vi "GUI - Copy.vi"() -> ()   [LabVIEW 2020]
uses:
  <vilib>/DAQmx/read.llb/DAQmx Read (Analog DBL 1Chan 1Samp).vi
  <vilib>/DAQmx/miscellaneous.llb/DAQmx Fill In Error Info.vi
  <vilib>/Utility/file.llb/Write Delimited Spreadsheet (string).vi
  <vilib>/Utility/file.llb/Write Delimited Spreadsheet (DBL).vi
  <vilib>/express/express arith-compare/Formula/XNode/ExpressFormulaBlockNode.xnode
panel:
  in  "stop":bool
  in  "Tab Control":enum32{"Overview", "Graphs"}(tab)
  out "NTU":dbl
  out "NTU":dbl
  out "NTU":dbl
  out "%":dbl
  out "L/s":dbl
  out "L/s":dbl
  in  "Gauge":bool
  in  "Coagulant Dose":bool
  in  "Switch":bool
  in  "Pump 2":bool
  in  "Pump 1":bool
  in  "UV254":bool
  in  "PID 3":bool
  in  "PID 2":bool
  in  "Valve 2":bool
  in  "Flow 2":bool
  in  "NTU 2":bool
  in  "NTU 3":bool
  in  "Flow 1":bool
  in  "Valve 1":bool
  in  "PID 1":bool
  in  "NTU 1":bool
  out "L/s":cluster{dbl[], dbl[]}[](graph)
  out "NTU":cluster{dbl[], dbl[]}[](graph)
  in  "Seconds per data point (sec)":dbl
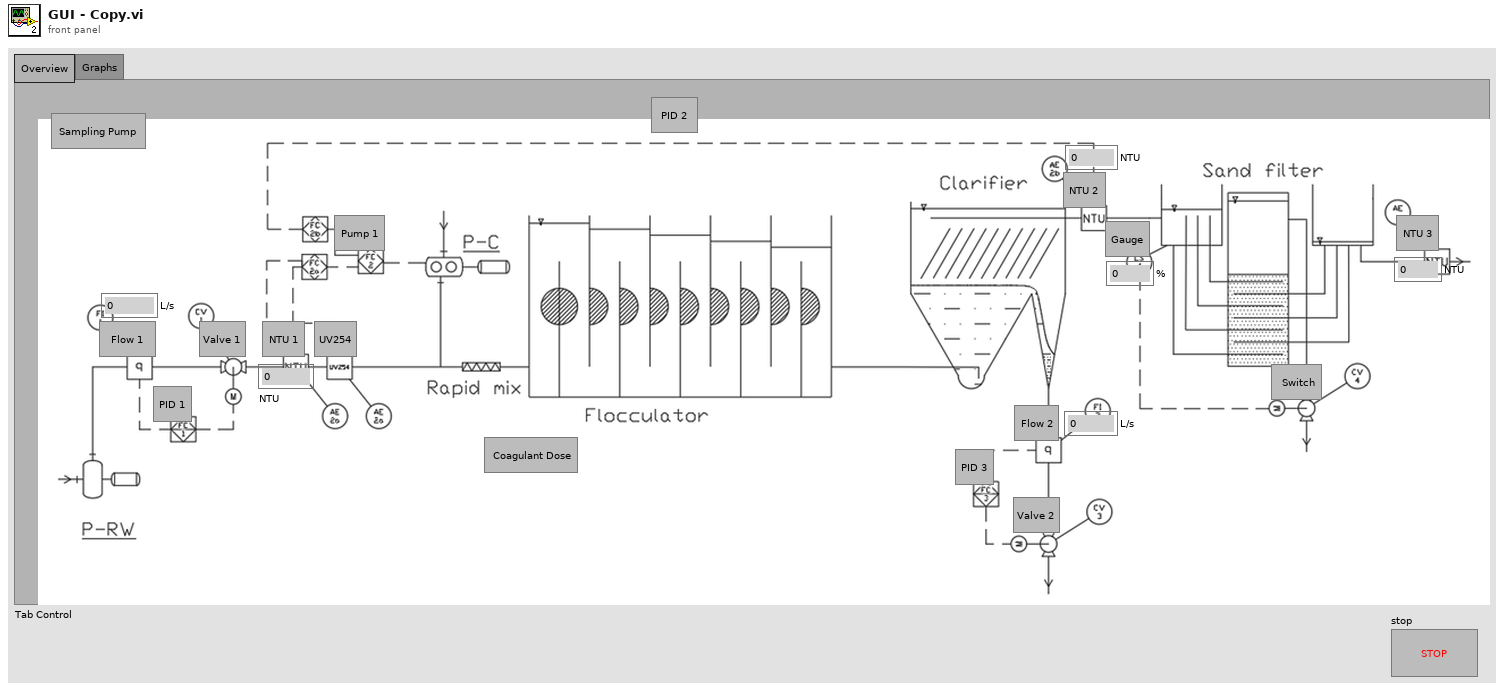
[diagram p1: front panel]
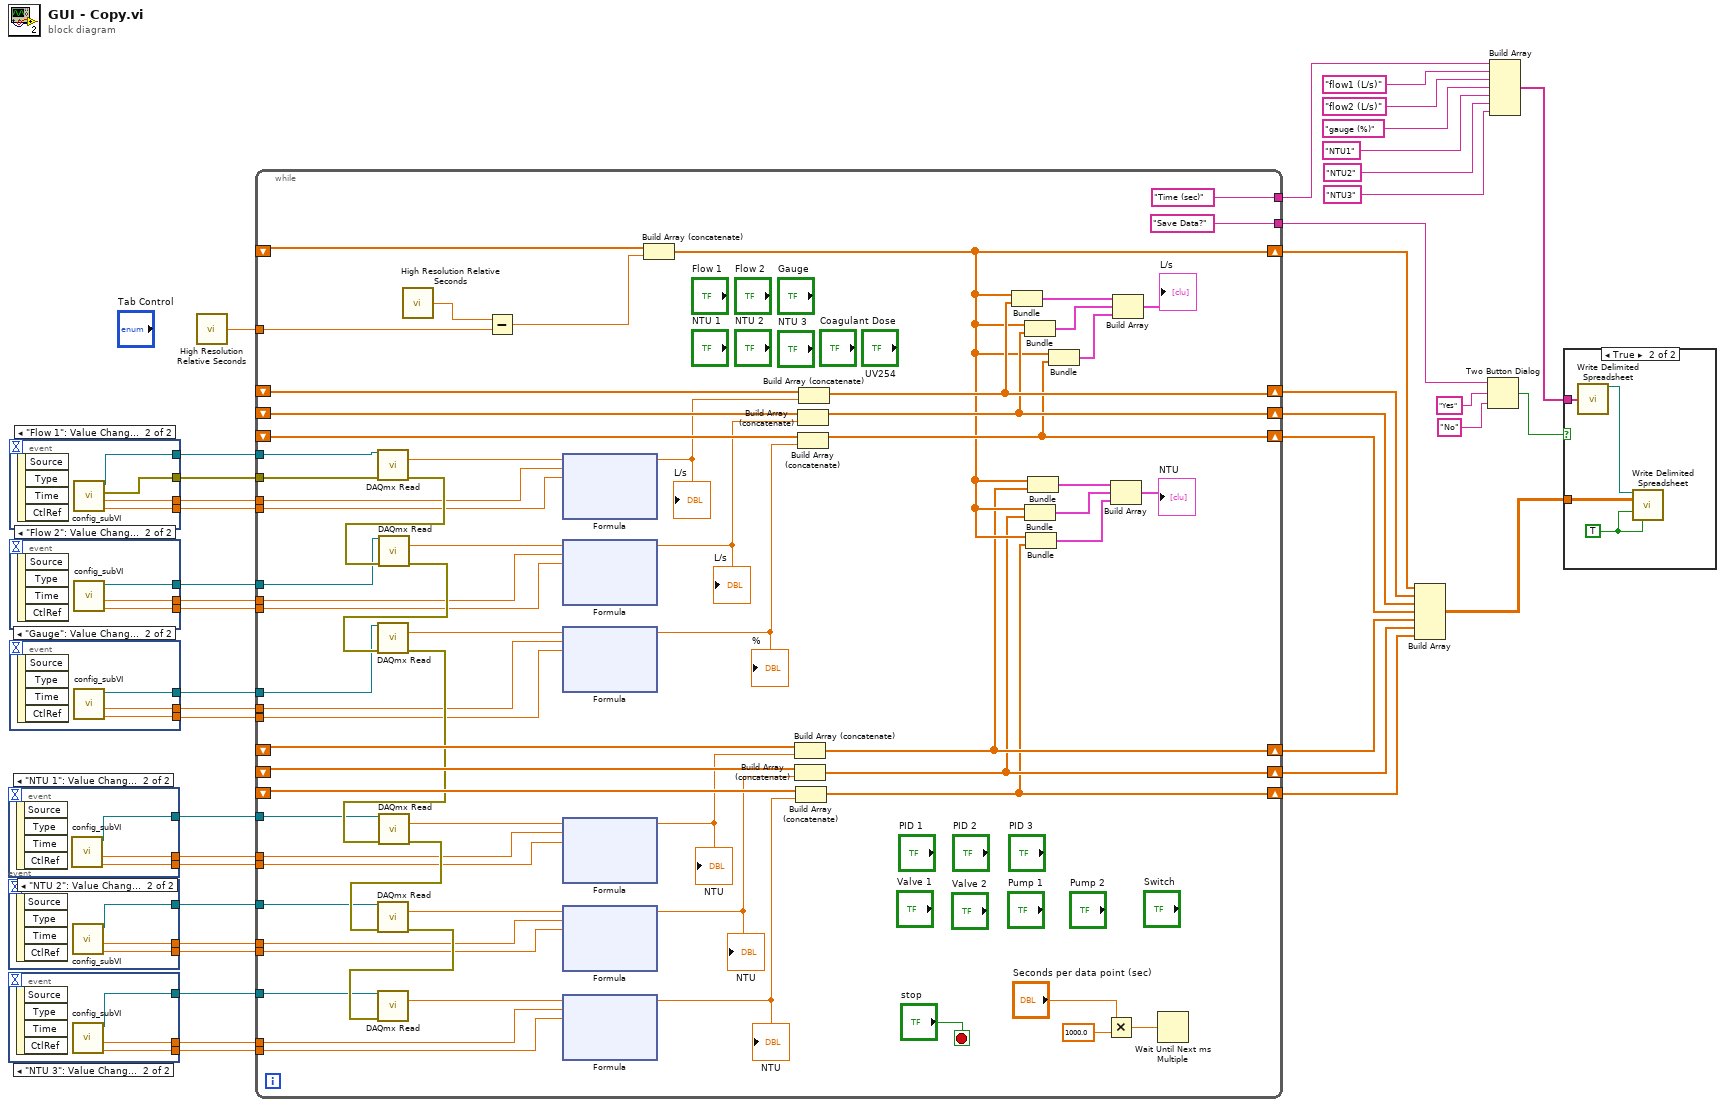
[diagram p0: block diagram]
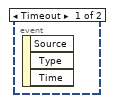
[diagram p3: hidden frame]
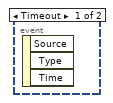
[diagram p4: hidden frame]
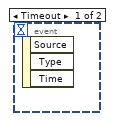
[diagram p5: hidden frame]
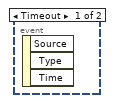
[diagram p6: hidden frame]
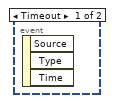
[diagram p7: hidden frame]
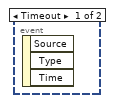
[diagram p8: hidden frame]
diagram:
  n1 = event shown="[1] \"NTU 1\": Value Change" {
    selector: _ -> [_ _]
    dyn-events: _ -> [_ _]
    timeout: _ -> [_ _]
    tunnel: [_ w43] -> w33
    tunnel: [_ w42] -> w32
    tunnel: [_ w41] -> w3
    event Timeout {
      n2 = event-data() -> ()  [unwired: 1 in, 3 out]
    }
    event "NTU 1": Value Change {
      n3 = event-data() -> ()  [unwired: 1 in, 4 out]
      n4 = call "config_subVI.vi"() -> ("B out"=w43:dbl, "A out"=w42:dbl, "task out"=w41:refnum<k21>)  [unwired: 8 in, 1 out]
    }
  }
  n5 = event shown="[1] \"NTU 2\": Value Change" {
    selector: _ -> [_ _]
    dyn-events: _ -> [_ _]
    timeout: _ -> [_ _]
    tunnel: [_ w46] -> w31
    tunnel: [_ w45] -> w30
    tunnel: [_ w44] -> w2
    event Timeout {
      n6 = event-data() -> ()  [unwired: 1 in, 3 out]
    }
    event "NTU 2": Value Change {
      n7 = event-data() -> ()  [unwired: 1 in, 4 out]
      n8 = call "config_subVI.vi"() -> ("B out"=w46:dbl, "A out"=w45:dbl, "task out"=w44:refnum<k21>)  [unwired: 8 in, 1 out]
    }
  }
  n9 = event shown="[1] \"NTU 3\": Value Change" {
    selector: _ -> [_ _]
    dyn-events: _ -> [_ _]
    timeout: _ -> [_ _]
    tunnel: [_ w49] -> w29
    tunnel: [_ w48] -> w28
    tunnel: [_ w47] -> w1
    event Timeout {
      n10 = event-data() -> ()  [unwired: 1 in, 3 out]
    }
    event "NTU 3": Value Change {
      n11 = event-data() -> ()  [unwired: 1 in, 4 out]
      n12 = call "config_subVI.vi"() -> ("B out"=w49:dbl, "A out"=w48:dbl, "task out"=w47:refnum<k21>)  [unwired: 8 in, 1 out]
    }
  }
  n13 = event shown="[1] \"Flow 1\": Value Change" {
    selector: _ -> [_ _]
    dyn-events: _ -> [_ _]
    timeout: _ -> [_ _]
    tunnel: [_ w53] -> w40
    tunnel: [_ w52] -> w39
    tunnel: [_ w51] -> w38
    tunnel: [_ w50] -> w6
    event Timeout {
      n14 = event-data() -> ()  [unwired: 1 in, 3 out]
    }
    event "Flow 1": Value Change {
      n15 = event-data() -> ()  [unwired: 1 in, 4 out]
      n16 = call "config_subVI.vi"() -> ("B out"=w53:dbl, "A out"=w52:dbl, "error out"=w51:errorcluster, "task out"=w50:refnum<k21>)  [unwired: 8 in]
    }
  }
  n17 = event shown="[1] \"Flow 2\": Value Change" {
    selector: _ -> [_ _]
    dyn-events: _ -> [_ _]
    timeout: _ -> [_ _]
    tunnel: [_ w56] -> w37
    tunnel: [_ w55] -> w36
    tunnel: [_ w54] -> w5
    event Timeout {
      n18 = event-data() -> ()  [unwired: 1 in, 3 out]
    }
    event "Flow 2": Value Change {
      n19 = event-data() -> ()  [unwired: 1 in, 4 out]
      n20 = call "config_subVI.vi"() -> ("B out"=w56:dbl, "A out"=w55:dbl, "task out"=w54:refnum<k21>)  [unwired: 8 in, 1 out]
    }
  }
  n21 = event shown="[1] \"Gauge\": Value Change" {
    selector: _ -> [_ _]
    dyn-events: _ -> [_ _]
    timeout: _ -> [_ _]
    tunnel: [_ w59] -> w35
    tunnel: [_ w58] -> w34
    tunnel: [_ w57] -> w4
    event Timeout {
      n22 = event-data() -> ()  [unwired: 1 in, 3 out]
    }
    event "Gauge": Value Change {
      n23 = event-data() -> ()  [unwired: 1 in, 4 out]
      n24 = call "config_subVI.vi"() -> ("B out"=w59:dbl, "A out"=w58:dbl, "task out"=w57:refnum<k21>)  [unwired: 8 in, 1 out]
    }
  }
  n25 = call <vilib>:"High Resolution Relative Seconds.vi"() -> ("relative seconds"=w7:dbl)
  n26 = while {
    shift-right: [w103] -> w27
    shift-left: _ -> [w123]
    shift-right: [w121] -> w26
    shift-left: _ -> [w122]
    shift-right: [w115] -> w25
    shift-left: _ -> [w116]
    shift-right: [w108] -> w24
    shift-left: _ -> [w109]
    shift-right: [w95] -> w21
    shift-left: _ -> [w98]
    shift-right: [w94] -> w22
    shift-left: _ -> [w97]
    shift-right: [w93] -> w23
    shift-left: _ -> [w96]
    tunnel: w40 -> [w81]
    tunnel: w39 -> [w80]
    tunnel: w38 -> [w79]
    tunnel: w37 -> [w78]
    tunnel: w36 -> [w77]
    tunnel: w35 -> [w76]
    tunnel: w34 -> [w75]
    tunnel: w33 -> [w74]
    tunnel: w32 -> [w73]
    tunnel: w31 -> [w72]
    tunnel: w30 -> [w71]
    tunnel: w29 -> [w66]
    tunnel: w28 -> [w70]
    tunnel: ["Time (sec)"] -> w20
    tunnel: ["Save Data?" ("message")] -> w13
    tunnel: w7 -> [w67]
    tunnel: w6 -> [w65]
    tunnel: w5 -> [w64]
    tunnel: w4 -> [w63]
    tunnel: w3 -> [w62]
    tunnel: w2 -> [w61]
    tunnel: w1 -> [w60]
    stop <- "stop" stop-if-true
    n27 = call-poly <vilib>:"DAQmx Read.vi"("task/channels in"=w65, "error in"=w79) -> ("data"=w106:dbl, "error out"=w86:errorcluster)  [unwired: 11 in, 1 out]
    n28 = call-poly <vilib>:"DAQmx Read.vi"("task/channels in"=w64, "error in"=w86) -> ("data"=w105:dbl, "error out"=w85:errorcluster)  [unwired: 11 in, 1 out]
    n29 = call-poly <vilib>:"DAQmx Read.vi"("task/channels in"=w63, "error in"=w85) -> ("data"=w104:dbl, "error out"=w84:errorcluster)  [unwired: 11 in, 1 out]
    n30 = call-poly <vilib>:"DAQmx Read.vi"("task/channels in"=w62, "error in"=w84) -> ("data"=w101:dbl, "error out"=w83:errorcluster)  [unwired: 11 in, 1 out]
    n31 = call-poly <vilib>:"DAQmx Read.vi"("task/channels in"=w61, "error in"=w83) -> ("data"=w100:dbl, "error out"=w82:errorcluster)  [unwired: 11 in, 1 out]
    n32 = call-poly <vilib>:"DAQmx Read.vi"("task/channels in"=w60, "error in"=w82) -> ("data"=w99:dbl)  [unwired: 11 in, 2 out]
    n33 = call <vilib>:"High Resolution Relative Seconds.vi"() -> ("relative seconds"=w125:dbl)
    n34 = Subtract(x=w125, y=w67) -> (x-y=w124:dbl)
    n35 = xnode "Formula"("data"=w106, "A"=w80, "B"=w81) -> ("Result"=w92:dbl)  [unwired: 1 in, 1 out]
    "L/s" <- w92
    n36 = xnode "Formula"("data"=w105, "A"=w77, "B"=w78) -> ("Result"=w91:dbl)  [unwired: 1 in, 1 out]
    "L/s" <- w91
    n37 = xnode "Formula"("data"=w104, "A"=w75, "B"=w76) -> ("Result"=w90:dbl)  [unwired: 1 in, 1 out]
    "%" <- w90
    n38 = xnode "Formula"("data"=w101, "A"=w73, "B"=w74) -> ("Result"=w87:dbl)  [unwired: 1 in, 1 out]
    "NTU" <- w87
    n39 = xnode "Formula"("data"=w100, "A"=w71, "B"=w72) -> ("Result"=w88:dbl)  [unwired: 1 in, 1 out]
    "NTU" <- w88
    n40 = xnode "Formula"("data"=w99, "A"=w70, "B"=w66) -> ("Result"=w89:dbl)  [unwired: 1 in, 1 out]
    "NTU" <- w89
    n41 = Build Array (concatenate)(w123, w124) -> (w103:dbl[])
    n42 = Build Array (concatenate)(w98, w87) -> (w95:dbl[])
    n43 = Build Array (concatenate)(w97, w88) -> (w94:dbl[])
    n44 = Build Array (concatenate)(w96, w89) -> (w93:dbl[])
    n45 = Build Array (concatenate)(w116, w91) -> (w115:dbl[])
    n46 = Build Array (concatenate)(w109, w90) -> (w108:dbl[])
    n47 = Build Array (concatenate)(w122, w92) -> (w121:dbl[])
    n48 = Bundle(w103, w121) -> (w120:cluster{dbl[], dbl[]})  [unwired: 1 in]
    n49 = Bundle(w103, w115) -> (w113:cluster{dbl[], dbl[]})  [unwired: 1 in]
    n50 = Bundle(w103, w94) -> (w110:cluster{dbl[], dbl[]})  [unwired: 1 in]
    n51 = Bundle(w103, w93) -> (w102:cluster{dbl[], dbl[]})  [unwired: 1 in]
    n52 = Bundle(w103, w95) -> (w111:cluster{dbl[], dbl[]})  [unwired: 1 in]
    n53 = Bundle(w103, w108) -> (w107:cluster{dbl[], dbl[]})  [unwired: 1 in]
    n54 = Multiply(x="Seconds per data point (sec)", y=1000.0) -> (x*y=w118:dbl)
    n55 = Build Array(w111, w110, w102) -> (→"NTU":cluster{dbl[], dbl[]}[])
    n56 = Build Array(w120, w113, w107) -> (→"L/s":cluster{dbl[], dbl[]}[])
    n57 = Wait Until Next ms Multiple(millisecond multiple=w118) -> ()  [unwired: 1 out]
  }
  n58 = Build Array(w27, w26, w25, w24, w21, w22, w23) -> (w8:dbl[][])
  n59 = Two Button Dialog(message=w13, 1:"No" ("F button name (\"Cancel\")"), 2:"Yes" ("T button name (\"OK\")")) -> (T button?=w9:bool)
  n60 = Build Array(w20, "flow1 (L/s)", "flow2 (L/s)", "gauge (%)", "NTU1", "NTU2", "NTU3") -> (w10:string[])
  n61 = case shown="True" w9 {
    tunnel: w8 -> [_ w202]
    tunnel: w10 -> [_ w201]
    frame False {
    }
    frame True {
      w199 = TRUE ("transpose? (no:F)")
      n62 = call-poly <vilib>:"Write Delimited Spreadsheet.vi"("1D data"=w201) -> ("new file path (Not A Path if cancelled)"=w200:path)  [unwired: 13 in, 1 out]
      n63 = call-poly <vilib>:"Write Delimited Spreadsheet.vi"("file path (dialog if empty)"=w200, "2D data"=w202, "append to file? (new file:F)"=w199, "transpose? (no:F)"=w199) -> ()  [unwired: 10 in, 2 out]
    }
  }
